vi "Set Initialization Data - Registration.vi"(8 "error in":errorcluster, 11 "gui in":refnum<class "gui.lvclass">) -> (0 "error out":errorcluster, 3 "gui out":refnum<class "gui.lvclass">)   [LabVIEW 2023, in "GUI.lvlib" / "gui.lvclass"]
doc: "In this VI you can set the initialization data of a statically-linked subWorker."
uses:
  gui.lvclass
  Registration Worker/Initialization Data.ctl
  Registration Worker/Response Cases.ctl
  <vilib>/addons/_Workers/Library/Case Label.ctl
  gui.lvclass/gui.ctl
  Registration Worker/Registration.lvclass
  C:/Program Files/National Instruments/LabVIEW 2023/vi.lib/addons/_Workers/Library/Classes/Worker/Worker.lvclass
  <vilib>/addons/_Workers/Library/Workers.lvlib
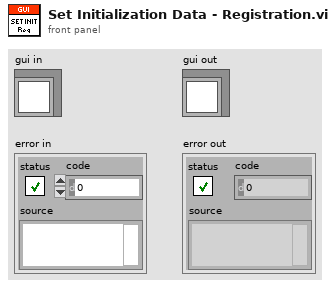
[diagram p1: front panel]
types:
  T1 = typedef "Registration.lvclass/Initialization Data.ctl" = cluster{"Response Cases":T2}
  T2 = typedef "Registration.lvclass/Response Cases.ctl" = cluster{"Placeholder - Can be deleted":string, "Record Status to Caller":T3}
  T3 = typedef "Workers.lvlib/Case Label.ctl" = string
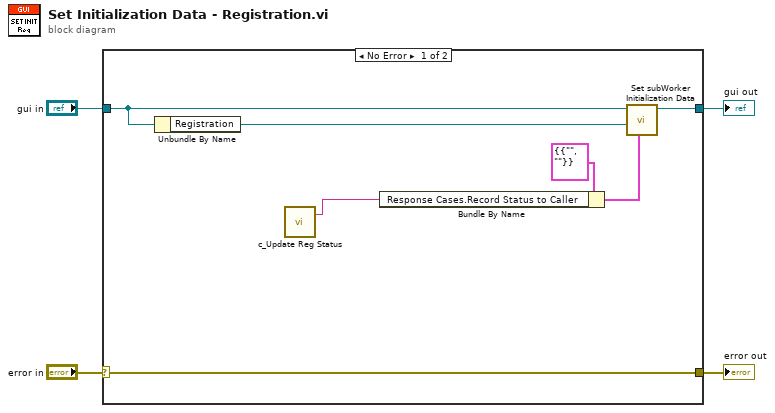
[diagram p0: block diagram]
diagram:
  n1 = case shown="No Error" "error in" {
    selector: "error in" -> [w11 w13]
    tunnel: [w11 w13] -> w3
    tunnel: [w9 w12] -> w2
    tunnel: "gui in" -> [w8 w12]
    frame No Error {
      n2 = Unbundle By Name(w8) -> ("Registration"=w10:refnum<class "Registration.lvclass">)
      n3 = call "c_Update Reg Status.vi"() -> ("Case Label"=w5:T3)  [unwired: 1 in]
      n4 = Bundle By Name(cluster=T1 {"Response Cases"={"Placeholder - Can be deleted"="", "Record Status to Caller"=""}} ("Initialization Data"), "Response Cases.Record Status to Caller"=w5) -> (w6:T1)
      n5 = call-dynamic "Set subWorker Initialization Data.vi"("Initialization Data"=w6, "subWorker"=w10, "Worker"=w8) -> ("Worker out"=w9:refnum<class "gui.lvclass">)  [unwired: 8 in]
    }
    frame Error {
    }
  }
  "error out" <- w3
  "gui out" <- w2
